vi "Format Cell Text Style.vi"(4 "Text Color (Unchanged)":u32(colorbox), 6 "BG Color (Unchanged)":u32(colorbox), 7 "Row Span (None)":i32, 8 "Error in":errorcluster caption="Error in (no error)", 10 "Text Alignment (Left)":T1="left", 11 "String":string) -> (0 "Error out":errorcluster, 3 "Formatted Text":string)   [LabVIEW 2023, in "Confluence Formatting.lvlib"]
uses:
  Confluence Formatting.lvlib
  Types/Text Alignment Combo Box.ctl
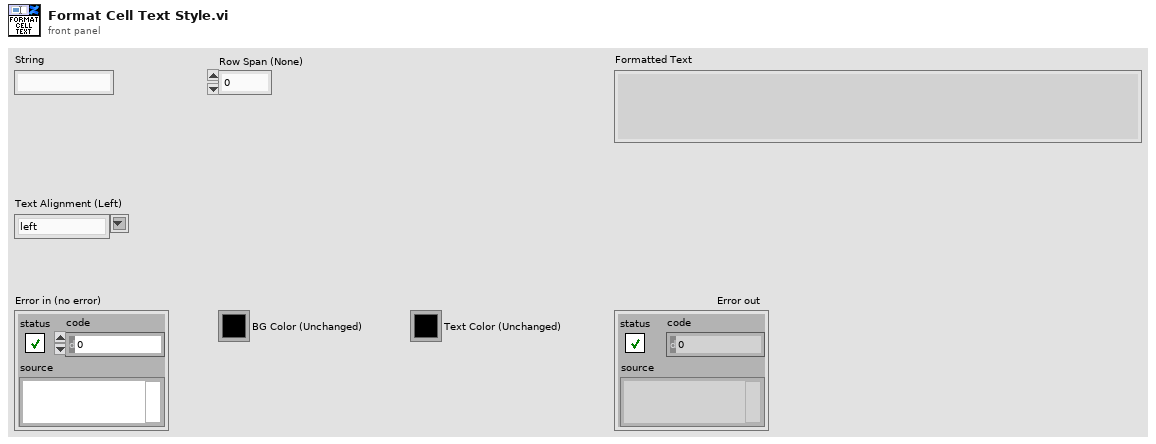
[diagram p1: front panel]
types:
  T1 = typedef "Confluence Formatting.lvlib/Text Alignment Combo Box.ctl" = string
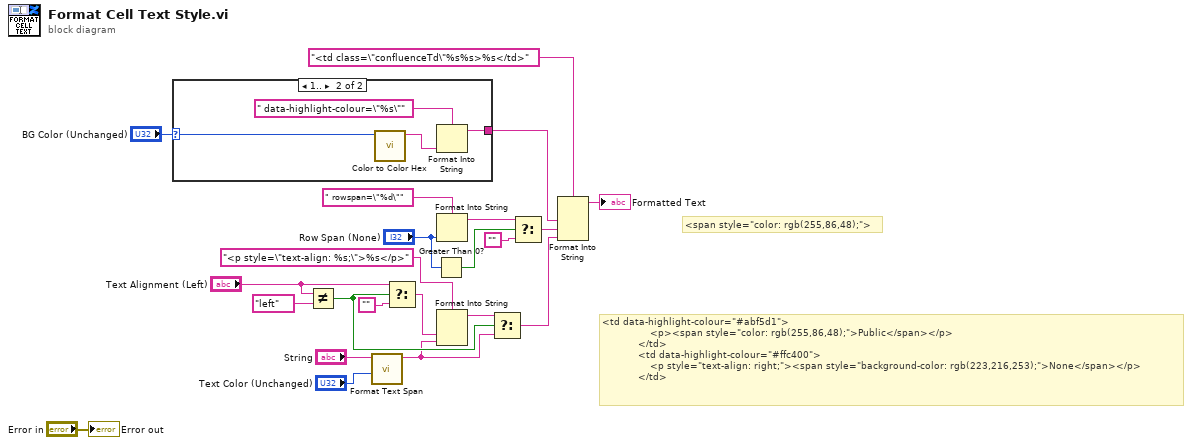
[diagram p0: block diagram]
diagram:
  # "<span style=\"color: rgb(255,86,48);\">"
  # "<td data-highlight-colour=\"#abf5d1\">\n                <p><span style=\"color: rgb(255,86,48);\">Public</span></p>\n            </td>\n            <td data-highlight-colour=\"#ffc400\">\n                <p style=\"text-align: right;\"><span style=\"background-color: rgb(223,216,253);\">None</span></p>\n            </td>"
  n1 = case shown="1.." "BG Color (Unchanged)" {
    selector: "BG Color (Unchanged)" -> [_ w24]
    tunnel: [_ w23] -> w9
    frame ..0 {
    }
    frame 1.. {
      n2 = call "Color to Color Hex.vi"("Color"=w24) -> ("Hex Color"=w25:string)  [unwired: 10 in]
      n3 = Format Into String(format string=" data-highlight-colour=\"%s\"", w25) -> (resulting string=w23:string)  [unwired: 2 in, 1 out]
    }
  }
  n4 = Not Equal?(x="Text Alignment (Left)", y=T1 "left") -> (x != y?=w12:bool)
  n5 = call "Format Text Span.vi"("Text Color (Unchanged)"="Text Color (Unchanged)", "Text"="String") -> ("Formatted Span"=w8:string)  [unwired: 8 in, 1 out]
  n6 = Select(t="Text Alignment (Left)", s=w12, f="") -> (s? t:f=w18:T1)
  n7 = Greater Than 0?(x="Row Span (None)") -> (x > 0?=w5:bool)
  n8 = Format Into String(format string=" rowspan=\"%d\"", "Row Span (None)") -> (resulting string=w2:string)  [unwired: 2 in, 1 out]
  n9 = Format Into String(format string="<p style=\"text-align: %s;\">%s</p>", w18, w8) -> (resulting string=w17:string)  [unwired: 2 in, 1 out]
  n10 = Select(t=w17, s=w12, f=w8) -> (s? t:f=w7:string)
  n11 = Select(t=w2, s=w5, f="") -> (s? t:f=w4:string)
  n12 = Format Into String(format string="<td class=\"confluenceTd\"%s%s>%s</td>", w9, w4, w7) -> (resulting string=→"Formatted Text":string)  [unwired: 2 in, 1 out]
  "Error out" <- "Error in"
